vi "Terminal-DAQ-6220-Getter.vi"(8 "error in (no error)":errorcluster caption="错误输入（无错误）", 10 "采样数(10)":i32=10, 11 "超时毫秒(5000)":i32=5000) -> (0 "error out":errorcluster caption="错误输出", 3 "6220":T1)   [LabVIEW 2014]
uses:
  Configuration-Global.vi
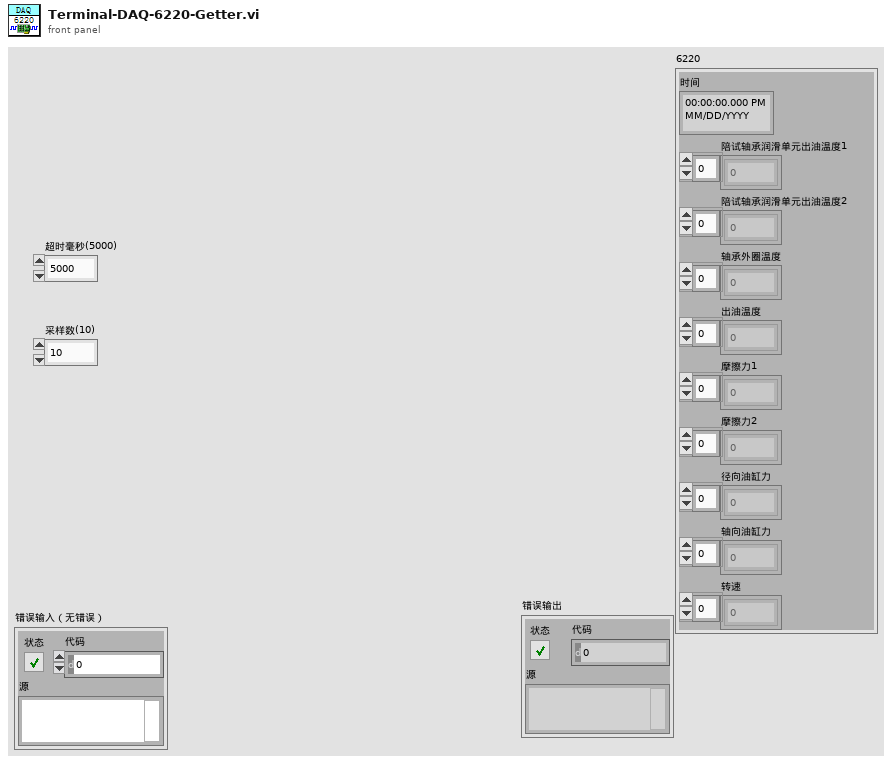
[diagram p1: front panel]
types:
  T1 = cluster{"时间":timestamp, "陪试轴承润滑单元出油温度1":sgl[], "陪试轴承润滑单元出油温度2":sgl[], "轴承外圈温度":sgl[], "出油温度":sgl[], "摩擦力1":sgl[], "摩擦力2":sgl[], "径向油缸力":sgl[], "轴向油缸力":sgl[], "转速":sgl[]}
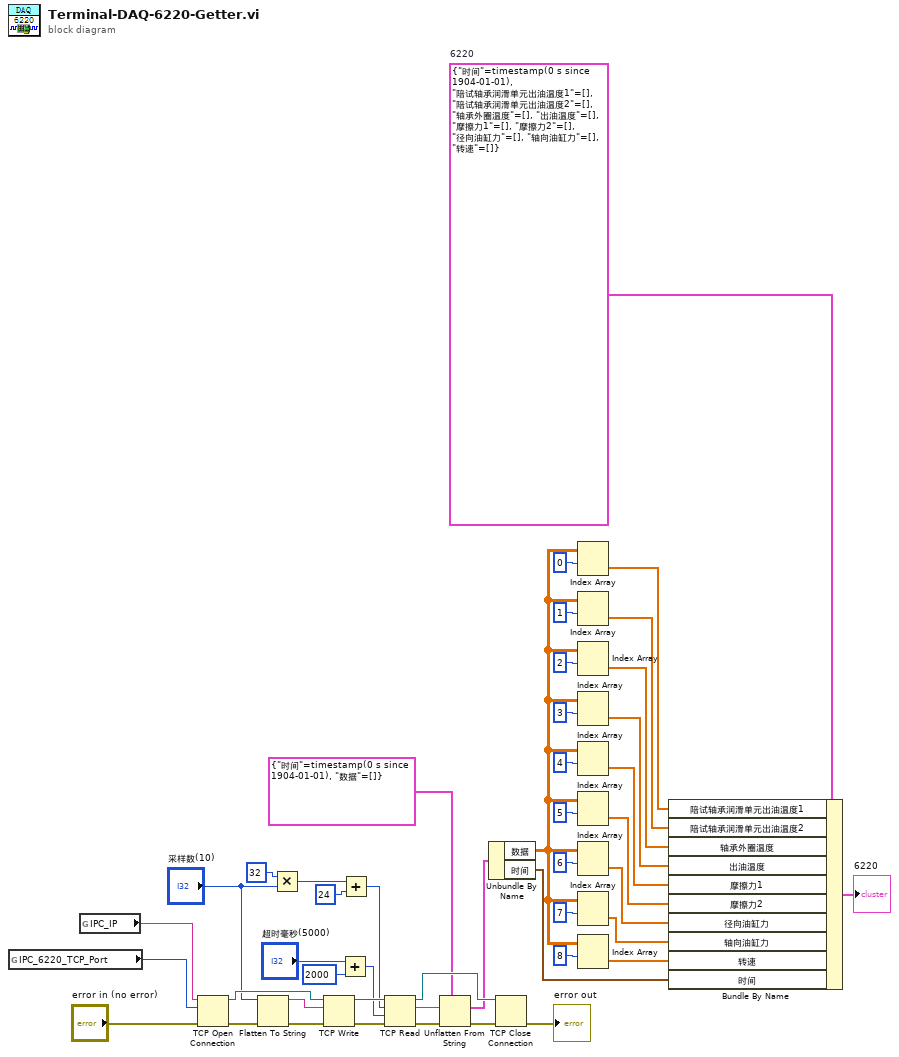
[diagram p0: block diagram]
diagram:
  w23 = T1 {"时间"=timestamp(0 s since 1904-01-01), "陪试轴承润滑单元出油温度1"=[], "陪试轴承润滑单元出油温度2"=[], "轴承外圈温度"=[], "出油温度"=[], "摩擦力1"=[], "摩擦力2"=[], "径向油缸力"=[], "轴向油缸力"=[], "转速"=[]}  # 6220
  n1 = global read "Configuration-Global.vi" "IPC_6220_TCP_Port"() -> (w2:i32)
  n2 = global read "Configuration-Global.vi" "IPC_IP"() -> (w1:string)
  n3 = TCP Open Connection(address=w1, remote port or service name=w2, error in (no error)="error in (no error)") -> (connection ID=w40:refnum<k5>, error out=w38:errorcluster)  [unwired: 2 in]
  n4 = Flatten To String(anything="采样数(10)", error in (no error)=w38) -> (data string=w36:string, error out=w37:errorcluster)  [unwired: 2 in, 1 out]
  n5 = Multiply(x=32, y="采样数(10)") -> (x*y=w8:i32)
  n6 = TCP Write(connection ID=w40, data in=w36, error in (no error)=w37) -> (connection ID out=w39:refnum<k5>, error out=w41:errorcluster)  [unwired: 1 in, 1 out]
  n7 = Add(x="超时毫秒(5000)", y=2000) -> (x+y=w3:i32)
  n8 = Add(x=w8, y=24) -> (x+y=w11:i32)
  n9 = TCP Read(connection ID=w39, bytes to read=w11, error in (no error)=w41, 9:w3) -> (connection ID out=w46:refnum<k5>, data out=w6:string, error out=w43:errorcluster)  [unwired: 1 in]
  n10 = Unflatten From String(type=cluster{"时间":timestamp, "数据":sgl[][]} {"时间"=timestamp(0 s since 1904-01-01), "数据"=[]}, binary string=w6, error in (no error)=w43) -> (value=w25:cluster{"时间":timestamp, "数据":sgl[][]}, error out=w42:errorcluster)  [unwired: 2 in, 1 out]
  n11 = Unbundle By Name(w25) -> ("数据"=w24:sgl[][], "时间"=w22:timestamp)
  n12 = TCP Close Connection(connection ID=w46, error in (no error)=w42) -> (error out=→"error out":errorcluster)  [unwired: 1 in, 1 out]
  n13 = Index Array(array=w24, index (row)=0 ("索引 (行)")) -> (element=w12:sgl[])  [unwired: 1 in]
  n14 = Index Array(array=w24, index (row)=1 ("索引 (行)")) -> (element=w21:sgl[])  [unwired: 1 in]
  n15 = Index Array(array=w24, index (row)=2 ("索引 (行)")) -> (element=w14:sgl[])  [unwired: 1 in]
  n16 = Index Array(array=w24, index (row)=3 ("索引 (行)")) -> (element=w15:sgl[])  [unwired: 1 in]
  n17 = Index Array(array=w24, index (row)=4 ("索引 (行)")) -> (element=w16:sgl[])  [unwired: 1 in]
  n18 = Index Array(array=w24, index (row)=5 ("索引 (行)")) -> (element=w17:sgl[])  [unwired: 1 in]
  n19 = Index Array(array=w24, index (row)=6 ("索引 (行)")) -> (element=w18:sgl[])  [unwired: 1 in]
  n20 = Index Array(array=w24, index (row)=7 ("索引 (行)")) -> (element=w19:sgl[])  [unwired: 1 in]
  n21 = Index Array(array=w24, index (row)=8 ("索引 (行)")) -> (element=w20:sgl[])  [unwired: 1 in]
  n22 = Bundle By Name(cluster=w23, "陪试轴承润滑单元出油温度1"=w12, "陪试轴承润滑单元出油温度2"=w21, "轴承外圈温度"=w14, "出油温度"=w15, "摩擦力1"=w16, "摩擦力2"=w17, "径向油缸力"=w18, "轴向油缸力"=w19, "转速"=w20, "时间"=w22) -> (→"6220":T1)
